vi "Abort.vi"(8 "error in (no error)":errorcluster, 11 "BuildWorker in":refnum<class "BuildWorker.lvclass">) -> (0 "error out":errorcluster, 3 "BuildWorker out":refnum<class "BuildWorker.lvclass">)   [LabVIEW 2017, in "BuildWorker.lvlib" / "BuildWorker.lvclass"]
uses:
  BuildWorker.lvclass
  Classes/Task/Status.ctl
  Classes/Task/Task.lvclass
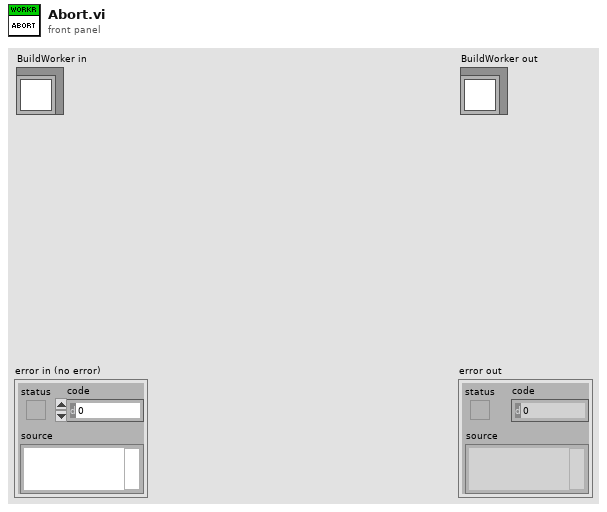
[diagram p1: front panel]
types:
  T1 = typedef "Task Interface.lvlib/Task.lvclass/Status.ctl" = enum16{"Created", "Added", "Pending", "Queued", "Processing", "Cleaning", "Building", "Finished", "Failed", "Removed", "Not found"}
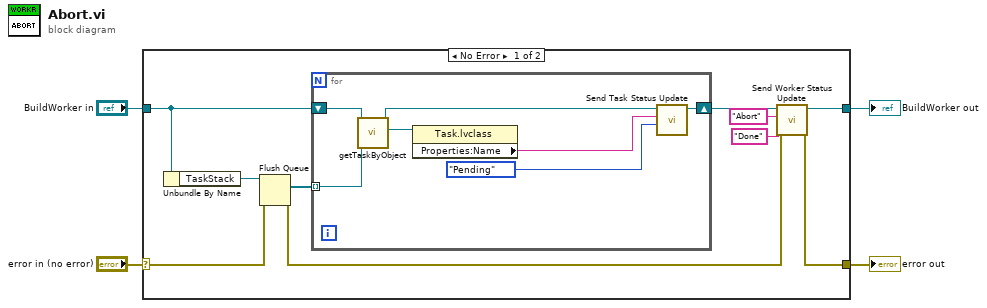
[diagram p0: block diagram]
diagram:
  n1 = case shown="No Error" "error in (no error)" {
    selector: "error in (no error)" -> [w13 w23]
    tunnel: [w7 w23] -> w3
    tunnel: [w9 w22] -> w1
    tunnel: "BuildWorker in" -> [w11 w22]
    frame No Error {
      n2 = Unbundle By Name(w11) -> ("TaskStack"=w14:refnum<queue>)
      n3 = Flush Queue(queue=w14, error in (no error)=w13) -> (remaining elements=w12:refnum<class "Task.lvclass">[], error out=w8:errorcluster)  [unwired: 1 out]
      n4 = for {
        tunnel: w12 -> [w20] mode=indexing
        shift-right: [w19] -> w10
        shift-left: w11 -> [w21]
        n5 = call "getTaskByObject.vi"("Task Object"=w20, "BuildWorker in"=w21) -> ("Task"=w16:refnum<class "Task.lvclass">, "BuildWorker out"=w17:refnum<class "BuildWorker.lvclass">)  [unwired: 7 in, 1 out]
        n6 = property class="Task.lvclass"(reference=w16) -> ("Properties:Name"=w15:string)  [unwired: 1 in, 2 out]
        n7 = call "Send Task Status Update.vi"("Status"=Status."Pending", "Task Name"=w15, "BuildWorker in"=w17) -> ("BuildWorker out"=w19:refnum<class "BuildWorker.lvclass">)  [unwired: 7 in, 1 out]
      }
      n8 = call "Send Worker Status Update.vi"("error in (no error)"=w8, "Status"="Done", "Operation"="Abort", "BuildWorker in"=w10) -> ("error out"=w7:errorcluster, "BuildWorker out"=w9:refnum<class "BuildWorker.lvclass">)  [unwired: 6 in]
    }
    frame Error {
    }
  }
  "error out" <- w3
  "BuildWorker out" <- w1
